vi "Day 3 task 2.vi"() -> ()   [LabVIEW 2022 SP3]
uses:
  fb686fa8-3d59-4615-83a8-50fde601e036.vi
  b9f48ee8-2cdb-4c23-9fb7-50a874023135.vi
  9099548b-f451-43ce-b1c0-cb01982e1de7.vi
  f26fad88-404b-46fb-af46-3f3a3c31c65f.vi
  <vilib>/Comparison/Less/Less Functor/Less Functor.lvclass
panel:
  out "string":string
  out "sum":u64
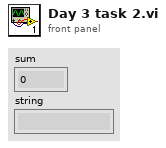
[diagram p1: front panel]
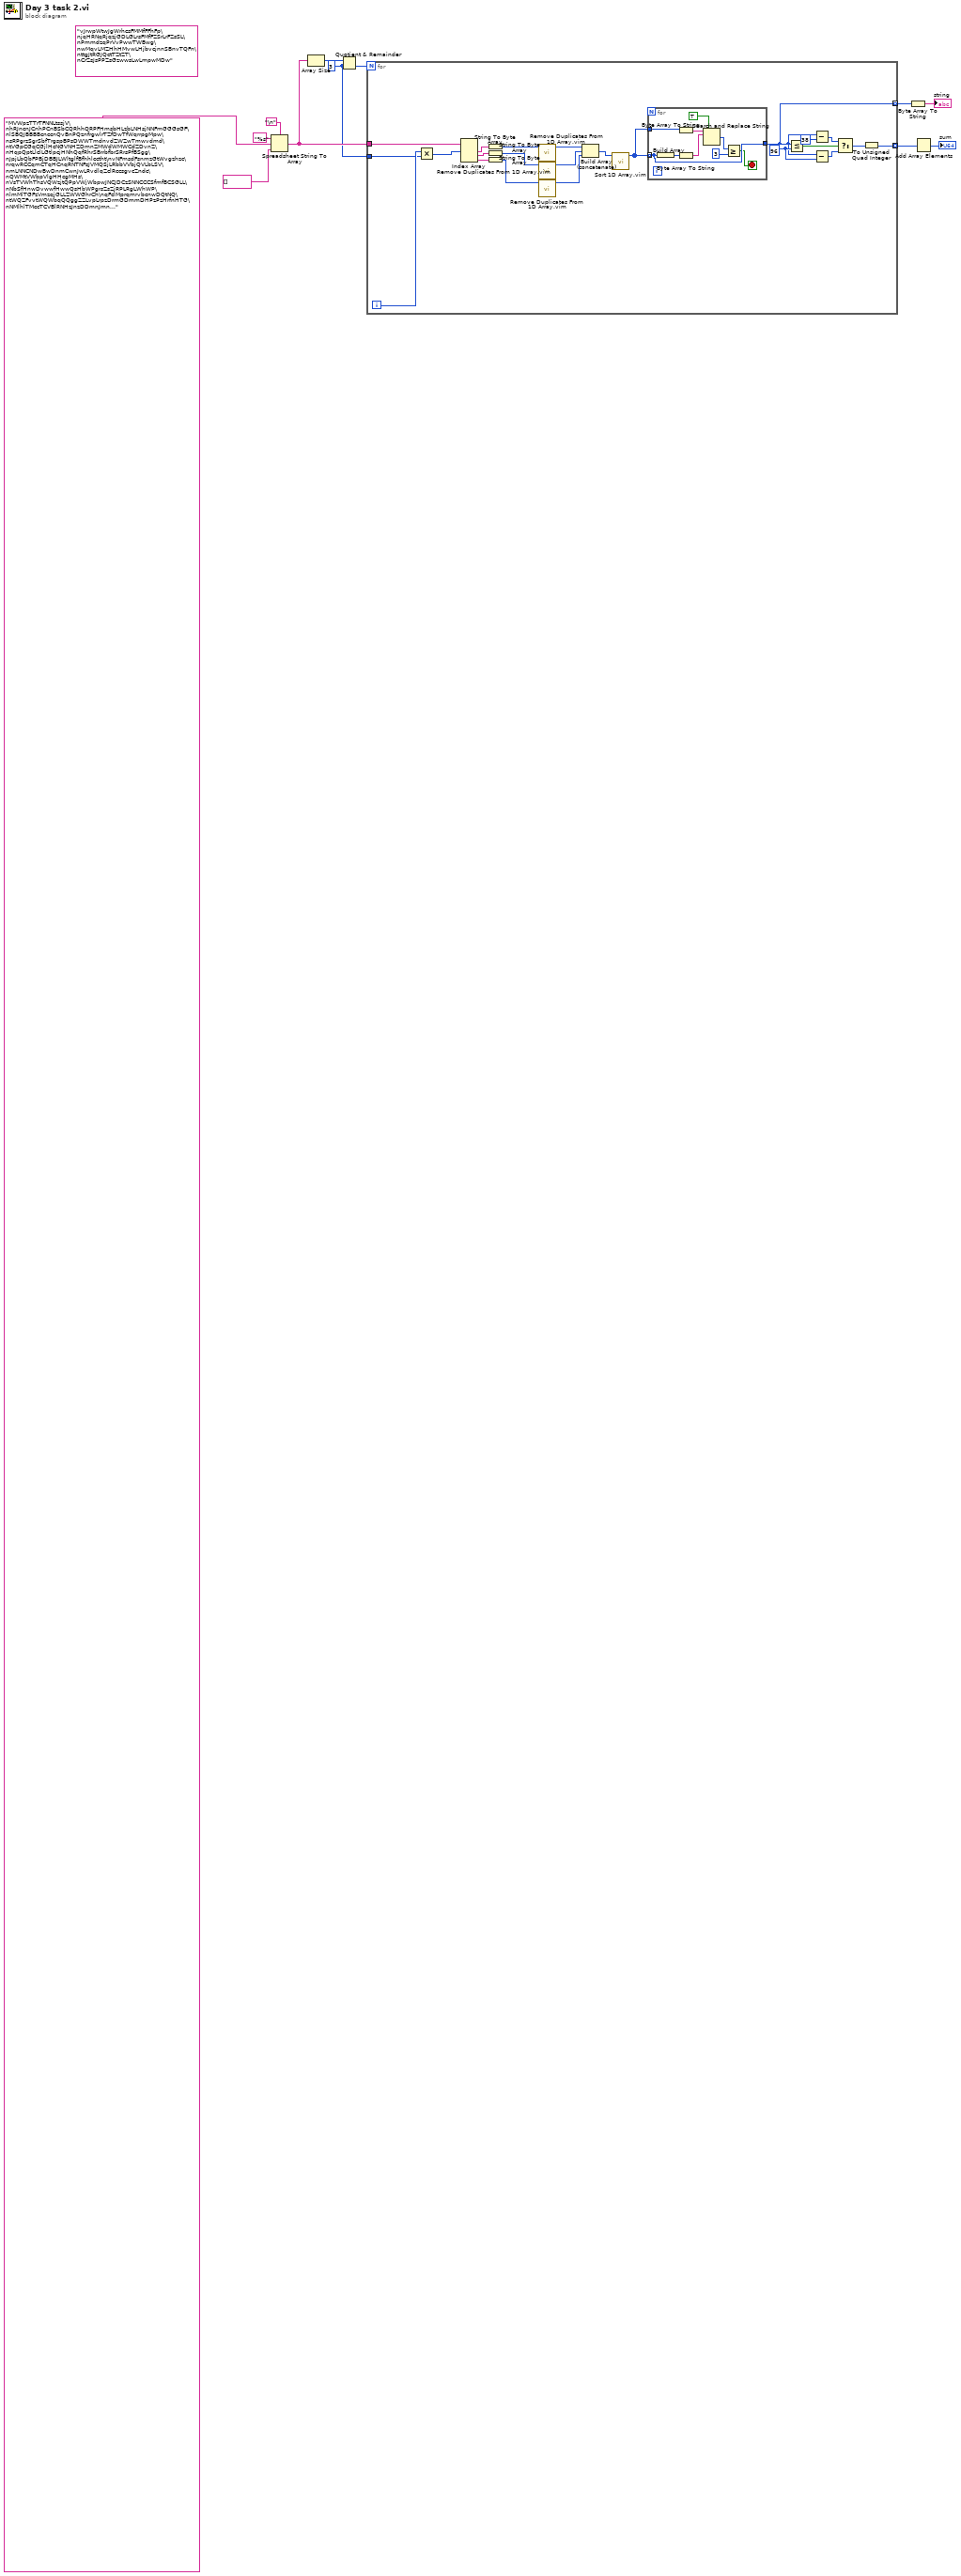
[diagram p0: block diagram]
diagram:
  w2 = 3 ("y")
  (unwired) "vJrwpWtwJgWrhcsFMMfFFhFp\njqHRNqRjqzjGDLGLrsFMfFZSrLrFZsSL\nPmmdzqPrVvPwwTWBwg\nwMqvLMZHhHMvwLHjbvcjnnSBnvTQFn\nttgJtRGJQctTZtZT\nCrZsJsPPZsGzwwsLwLmpwMDw"
  n1 = Spreadsheet String To Array(delimiter (Tab)="\n", format string="%s", spreadsheet string="MVWpzTTrTFNNLtssjV\nhRJncnJCnhPCnBSbCQRhhQRPFHmsbHLzbLNHsjNNFmGGGsGF\nlSBQJBBBBcnccnQvBnPQznfrgwlrTZfDwTfWqrrpgMpw\nsRPgrzSgrSbfTrgspBPsDWWTmdnvdZWZwTmwvdmd\ntVGpCGqCGjlHcNGVNHZDmnZMWdWMWCdZDvnZ\nHqpQptLlclLGtlpcjHNhQqfRhrSBrrbfbrSRrsPfBSgg\nJpjLbQbFPBjDBBJLWltglfBfhhlcctht\nvNFmsdFsnmzGtWvgzhzc\nrqwRCCqmCTqHCnqRNTNFsJVMQSjLRbbVVbjQVLbLSV\nmLNNCNDwBwDnmCwnJwLRvdlqZclRccsgvcZndc\nQWMtVWbpVlgHHcgMHs\nVsTVWhThsVQWzjtQPpVWjWbpwJNCJDCzSNNCCCSfmfBCSGLL\nNbSfHnwDvwwfHwwQsHbWPgrsZsZjRPLRgLWhWP\nlmMlTGFzVmzqjGLLZWWGhrCh\nqFclMprqmrvbcnwDQtNQ\ntWQZFvvtWQWbqQQggZZLvpLrpzDrmGDmmDHPzPzHrfnHTG\nNMlhlTMccTCVBlRNHzJnzDDmnJmn...", array type (2D Dbl)=string[] [] ("format string")) -> (array=w6:string[])
  n2 = Array Size(array=w6) -> (size(s)=w8:i32)
  n3 = Quotient & Remainder(x=w8, y=w2) -> (floor(x/y)=w7:i32)  [unwired: 1 out]
  n4 = for {
    N: w7 -> [_]
    tunnel: [w24] -> w5 mode=indexing
    tunnel: w6 -> [w35]
    tunnel: [w23] -> w4 mode=indexing
    tunnel: w2 -> [w20]
    i -> [w22]
    w26 = u8 96 ("y")
    n5 = Multiply(x=w22, y=w20) -> (x*y=w21:i32)
    n6 = Index Array(array=w35, index #1=w21) -> (element #1=w34:string, element #2=w33:string, element #3=w32:string)  [unwired: 2 in]
    n7 = String To Byte Array(string=w34) -> (unsigned byte array=w19:u8[])
    n8 = String To Byte Array(string=w33) -> (unsigned byte array=w17:u8[])
    n9 = String To Byte Array(string=w32) -> (unsigned byte array=w16:u8[])
    n10 = call "Remove Duplicates From 1D Array.vim"("array"=w19) -> ("array with duplicates removed"=w18:u8[])  [unwired: 10 in]
    n11 = call "Remove Duplicates From 1D Array.vim"("array"=w17) -> ("array with duplicates removed"=w15:u8[])  [unwired: 10 in]
    n12 = call "Remove Duplicates From 1D Array.vim"("array"=w16) -> ("array with duplicates removed"=w14:u8[])  [unwired: 10 in]
    n13 = Build Array (concatenate)(w18, w15, w14) -> (w31:u8[])
    n14 = call "Sort 1D Array.vim"("unsorted array"=w31) -> ("sorted array"=w13:u8[])  [unwired: 10 in]
    n15 = for {
      tunnel: w13 -> [w39] mode=indexing
      tunnel: [w39] -> w23
      tunnel: w13 -> [w42]
      stop <- w36 stop-if-true
      n16 = Build Array(w39) -> (w43:u8[])
      n17 = Byte Array To String(unsigned byte array=w42) -> (string=w41:string)
      n18 = Byte Array To String(unsigned byte array=w43) -> (string=w44:string)
      n19 = Search and Replace String(replace all?=TRUE ("replace all? (F)"), input string=w41, search string=w44) -> (number of replacements=w38:i32)  [unwired: 5 in, 3 out]
      n20 = Greater Or Equal?(x=w38, y=3) -> (x >= y?=w36:bool)
    }
    n21 = Less Or Equal?(x=w23, y=w26) -> (x <= y?=w30:bool)
    n22 = Subtract(x=w23, y=u8 38) -> (x-y=w28:u8)
    n23 = Subtract(x=w23, y=w26) -> (x-y=w29:u8)
    n24 = Select(t=w28, s=w30, f=w29) -> (s? t:f=w25:u8)
    n25 = To Unsigned Quad Integer(1:w25) -> (0:w24:u64)
  }
  n26 = Byte Array To String(unsigned byte array=w4) -> (string=→"string":string)
  n27 = Add Array Elements(numeric array=w5) -> (sum=→"sum":u64)
